vi "Set_Control_Values_by_Index_(Sgnl) for Lamps.vi"(7 "Control References":refnum<vi>[](array[refnum]), 8 "error in (no error)":errorcluster, 9 "appended array":variant[](array[variant])) -> (0 "error out":errorcluster)   [LabVIEW 2015]
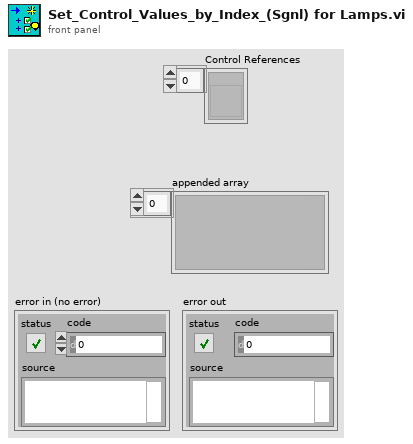
[diagram p1: front panel]
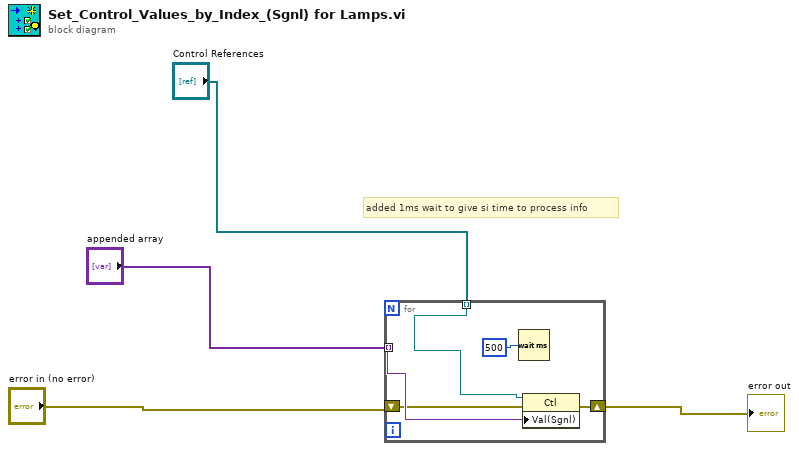
[diagram p0: block diagram]
diagram:
  # "added 1ms wait to give si time to process info"
  n1 = for {
    shift-right: [w9] -> w4
    shift-left: "error in (no error)" -> [w6]
    tunnel: "Control References" -> [w8] mode=indexing
    tunnel: "appended array" -> [w7] mode=indexing
    n2 = Wait (ms)(milliseconds to wait=500) -> ()  [unwired: 1 out]
    n3 = property class="Ctl"(reference=w8, error in=w6, "Val(Sgnl)"=w7) -> (error out=w9:errorcluster)  [unwired: 1 out]
  }
  "error out" <- w4
